vi "close_tasks.vi"(0 "Counter (in)":refnum<class "Counter.lvclass">, 1 "HSDIO (in)":refnum<class "HSDIO.lvclass">, 2 "Camera (in)":refnum<class "Camera.lvclass">, 3 "TTL_input in":refnum<class "TTL_input.lvclass">, 5 "error in":errorcluster) -> (14 "Counter":refnum<class "Counter.lvclass">, 15 "HSDIO":refnum<class "HSDIO.lvclass">, 16 "Camera":refnum<class "Camera.lvclass">, 17 "TTL_input out":refnum<class "TTL_input.lvclass">, 19 "error out":errorcluster)   [LabVIEW 2013]
uses:
  HSDIO/HSDIO.lvclass
  Camera/Camera.lvclass
  Counter/Counter.lvclass
  TTL_input/TTL_input.lvclass
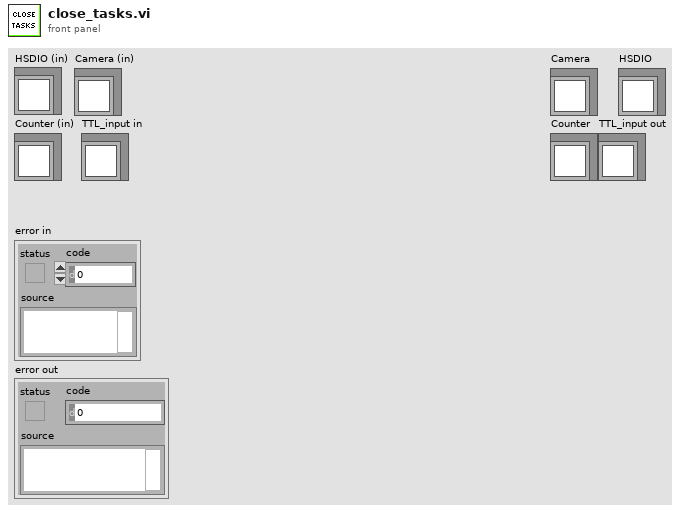
[diagram p1: front panel]
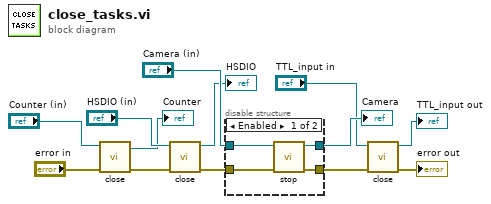
[diagram p0: block diagram]
diagram:
  n1 = call-dynamic "close.vi"("error in (no error)"="error in", "Counter in"="Counter (in)") -> ("error out"=w6:errorcluster, "Counter out"=→"Counter":refnum<class "Counter.lvclass">)  [unwired: 8 in]
  n2 = call-dynamic "close.vi"("error in (no error)"=w6, "HSDIO in"="HSDIO (in)") -> ("error out"=w12:errorcluster, "HSDIO out"=→"HSDIO":refnum<class "HSDIO.lvclass">)  [unwired: 8 in]
  n3 = disable-structure shown="Enabled" {
    disable-tunnel: w12 -> [w17 w18]
    disable-tunnel: [w16 w18] -> w3
    disable-tunnel: "Camera (in)" -> [w15 w19]
    disable-tunnel: [w14 w19] -> w10
    frame Enabled {
      n4 = call-dynamic "stop.vi"("error in (no error)"=w17, "Camera in"=w15) -> ("error out"=w16:errorcluster, "Camera out"=w14:refnum<class "Camera.lvclass">)  [unwired: 8 in]
    }
    frame Disabled {
    }
  }
  "Camera" <- w10
  n5 = call-dynamic "close.vi"("error in (no error)"=w3, "TTL_input in"="TTL_input in") -> ("error out"=→"error out":errorcluster, "TTL_input out"=→"TTL_input out":refnum<class "TTL_input.lvclass">)  [unwired: 8 in]
